vi "FGEN Output Enable.vi"(8 "error in (no error)":errorcluster, 10 "Output Enable (default: True)":bool=TRUE, 11 "Function Generator in":refnum<class "Function Generator.lvclass">) -> (0 "error out":errorcluster, 3 "Function Generator out":refnum<class "Function Generator.lvclass">)   [LabVIEW 2023, in "HardwareAbstractionLayer_LVOOP.lvlib" / "Function Generator.lvclass"]
uses:
  Function Generator.lvclass
  Function Generator.lvclass/Function Generator.ctl
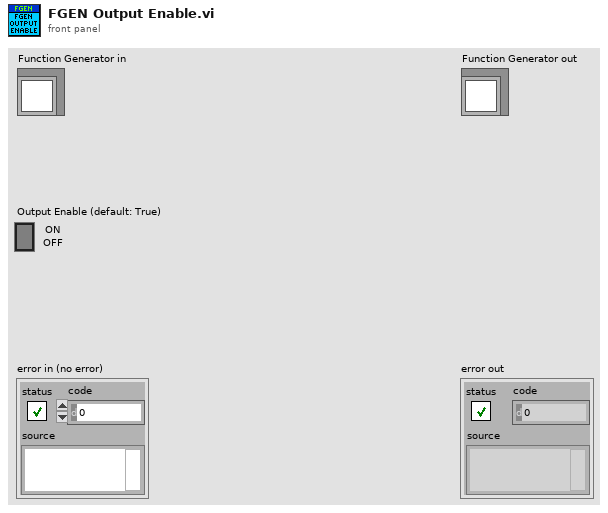
[diagram p1: front panel]
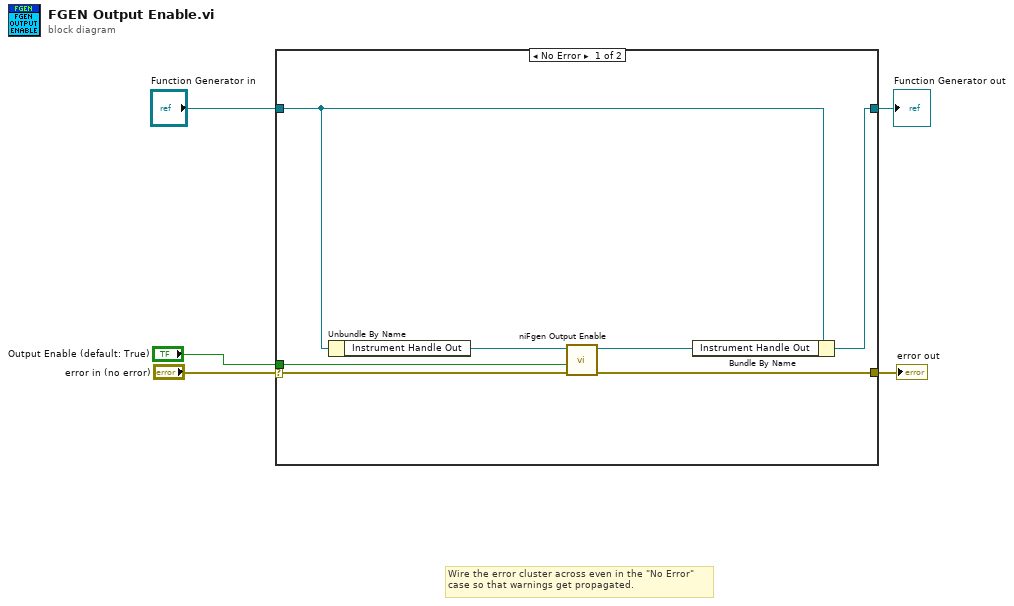
[diagram p0: block diagram]
diagram:
  # "Wire the error cluster across even in the \"No Error\"\ncase so that warnings get propagated."
  n1 = case shown="No Error" "error in (no error)" {
    selector: "error in (no error)" -> [w12 w14]
    tunnel: [w11 w14] -> w4
    tunnel: [w7 w13] -> w2
    tunnel: "Function Generator in" -> [w8 w13]
    tunnel: "Output Enable (default: True)" -> [w10 _]
    frame No Error {
      n2 = Unbundle By Name(w8) -> ("Instrument Handle Out"=w9:refnum<k15>)
      n3 = call <instrlib>:"niFgen Output Enable.vi"("error in (no error)"=w12, "Output Enable (default: True)"=w10, "Instrument Handle"=w9) -> ("error out"=w11:errorcluster, "Instrument Handle Out"=w6:refnum<k15>)  [unwired: 7 in]
      n4 = Bundle By Name(cluster=w8, "Instrument Handle Out"=w6) -> (w7:refnum<class "Function Generator.lvclass">)
    }
    frame Error {
    }
  }
  "error out" <- w4
  "Function Generator out" <- w2
